vi "icsTest.vi"() -> ()   [LabVIEW 2014]
panel:
  in  "Stop":bool
  in  "Cancel":bool
  in  "Steps 1":i32
  in  "Config 1":string="{0:1,2:-1}"
  in  "OK":bool
  in  "Steps 0":i32
  in  "Config 0":string="{0:1,2:1}"
  out "Vact 3":dbl=1.0 format="%.1f"
  in  "Vset 3":dbl=1.0 format="%.1f"
  out "Vact 2":dbl=1.0 format="%.1f"
  in  "Vset 2":dbl=1.0 format="%.1f"
  out "Vact 1":dbl=1.0 format="%.1f"
  in  "Vset 1":dbl=1.0 format="%.1f"
  out "Vact 0":dbl=1.0 format="%.1f"
  in  "Parameter":u16(ring) items=["Frequency (MHz)", "Amplitude (dBm)", "Phase (Pi)"]
  in  "Vset 0":dbl=1.0 format="%.1f"
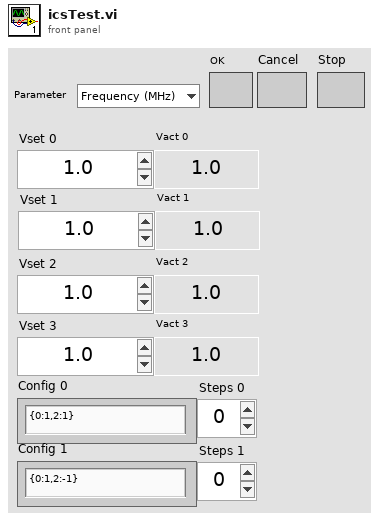
[diagram p1: front panel]
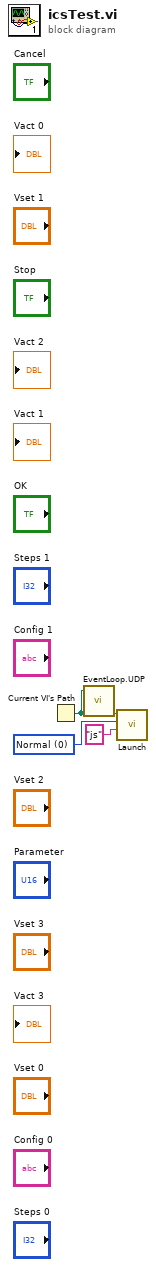
[diagram p0: block diagram]
diagram:
  w1 = u16 0 items=["Normal", "Keep", "Hide"] ("Mode")
  n1 = Current VI's Path() -> (path=w3:path)
  n2 = call "EventLoop.UDP.vi"("Path"=w3) -> ()  [unwired: 2 in]
  n3 = call "Launch.vi"("Cmd"="js", "Mode"=w1, "Path"=w3) -> ()  [unwired: 1 in]
